vi "Get Channel Value by Data Reference.vi"(8 "error in":errorcluster, 10 "Data Reference in":i32, 11 "Custom Device API in":refnum<class "Custom Device API.lvclass">) -> (0 "error out":errorcluster, 2 "Value":dbl, 3 "Custom Device API out":refnum<class "Custom Device API.lvclass">)   [LabVIEW 2027, in "Custom Device Interfaces.lvlib" / "Custom Device API.lvclass"]
uses:
  Custom Device API.lvclass
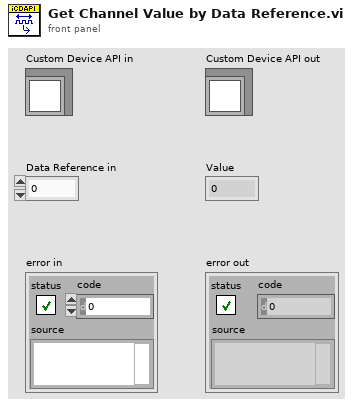
[diagram p1: front panel]
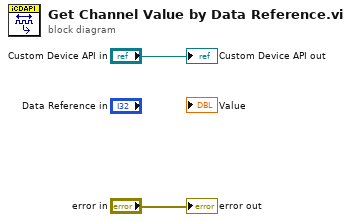
[diagram p0: block diagram]
diagram:
  "error out" <- "error in"
  "Custom Device API out" <- "Custom Device API in"
